vi "ConvertHexDataToHexString.vi"(11 "hex data(not string)":string) -> (3 "string-hex":string)   [LabVIEW 2018]
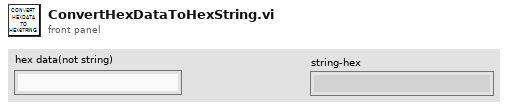
[diagram p1: front panel]
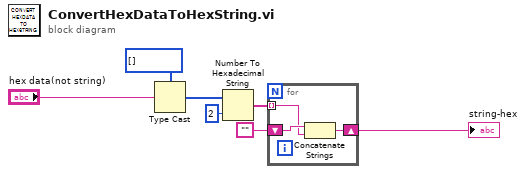
[diagram p0: block diagram]
diagram:
  n1 = Type Cast(type=i8[] [], x="hex data(not string)") -> (*(type *) &x=w3:i8[])
  n2 = Number To Hexadecimal String(1:i16 2 ("폭(-)"), 2:w3) -> (0:w7:string[])
  n3 = for {
    tunnel: w7 -> [w8] mode=indexing
    shift-right: [w10] -> w1
    shift-left: "" -> [w9]
    n4 = Concatenate Strings(w9, w8) -> (w10:string)
  }
  "string-hex" <- w1
